vi "Main.vi"() -> ()   [LabVIEW 2014]
uses:
  Goomba Direction.ctl
panel:
  out "Time":i32
  out "Score":i32
  in  "?":bool
  out "?":picture
  in  "Start Game":bool
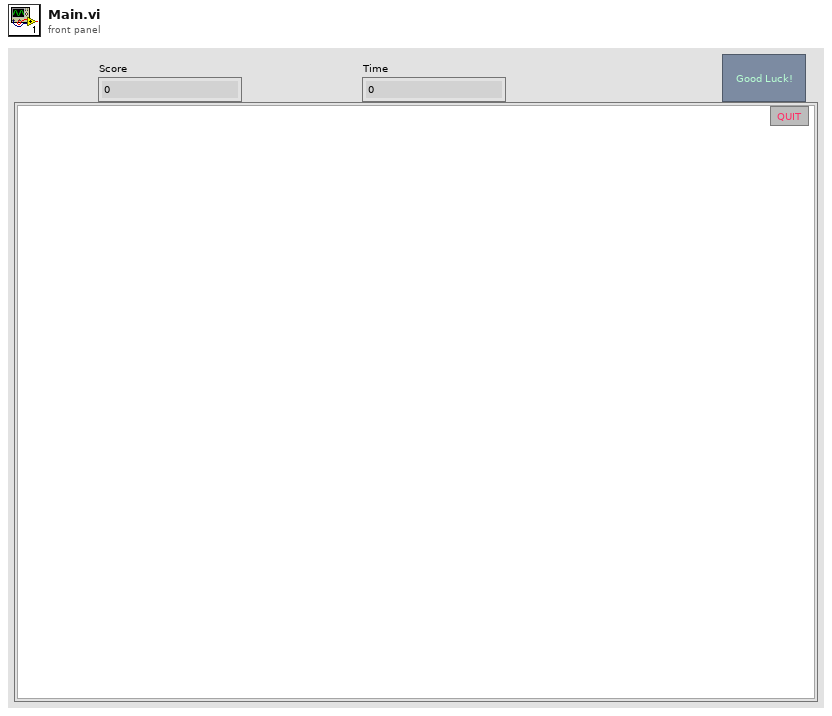
[diagram p1: front panel]
types:
  T1 = typedef "Goomba Direction.ctl" = enum16{"Left", "Right"}
  T2 = typedef "eventvkey.ctl" = enum16{"ASCII", "Enter", "Return", "Shift", "Ctrl", "Alt", "Cmd", "Opt", "Caps", "NumLock", "Clear", "Break", "Up", "Down", "Left", "Right", "Insert", "Delete", "Home", "End", "PageUp", "PageDown", "Escape", "Help", "Pause", "ScrollLock", "F1", "F2", "F3", "F4", "F5", "F6", "F7", "F8", "F9", "F10", "F11", "F12", "F13", "F14", "F15", "F16", "F17", "F18", "F19", "F20", "F21", "F22", "F23", "F24", "Play", "VolumeUp", "VolumeDown", "Mute", "Two Byte Char"}
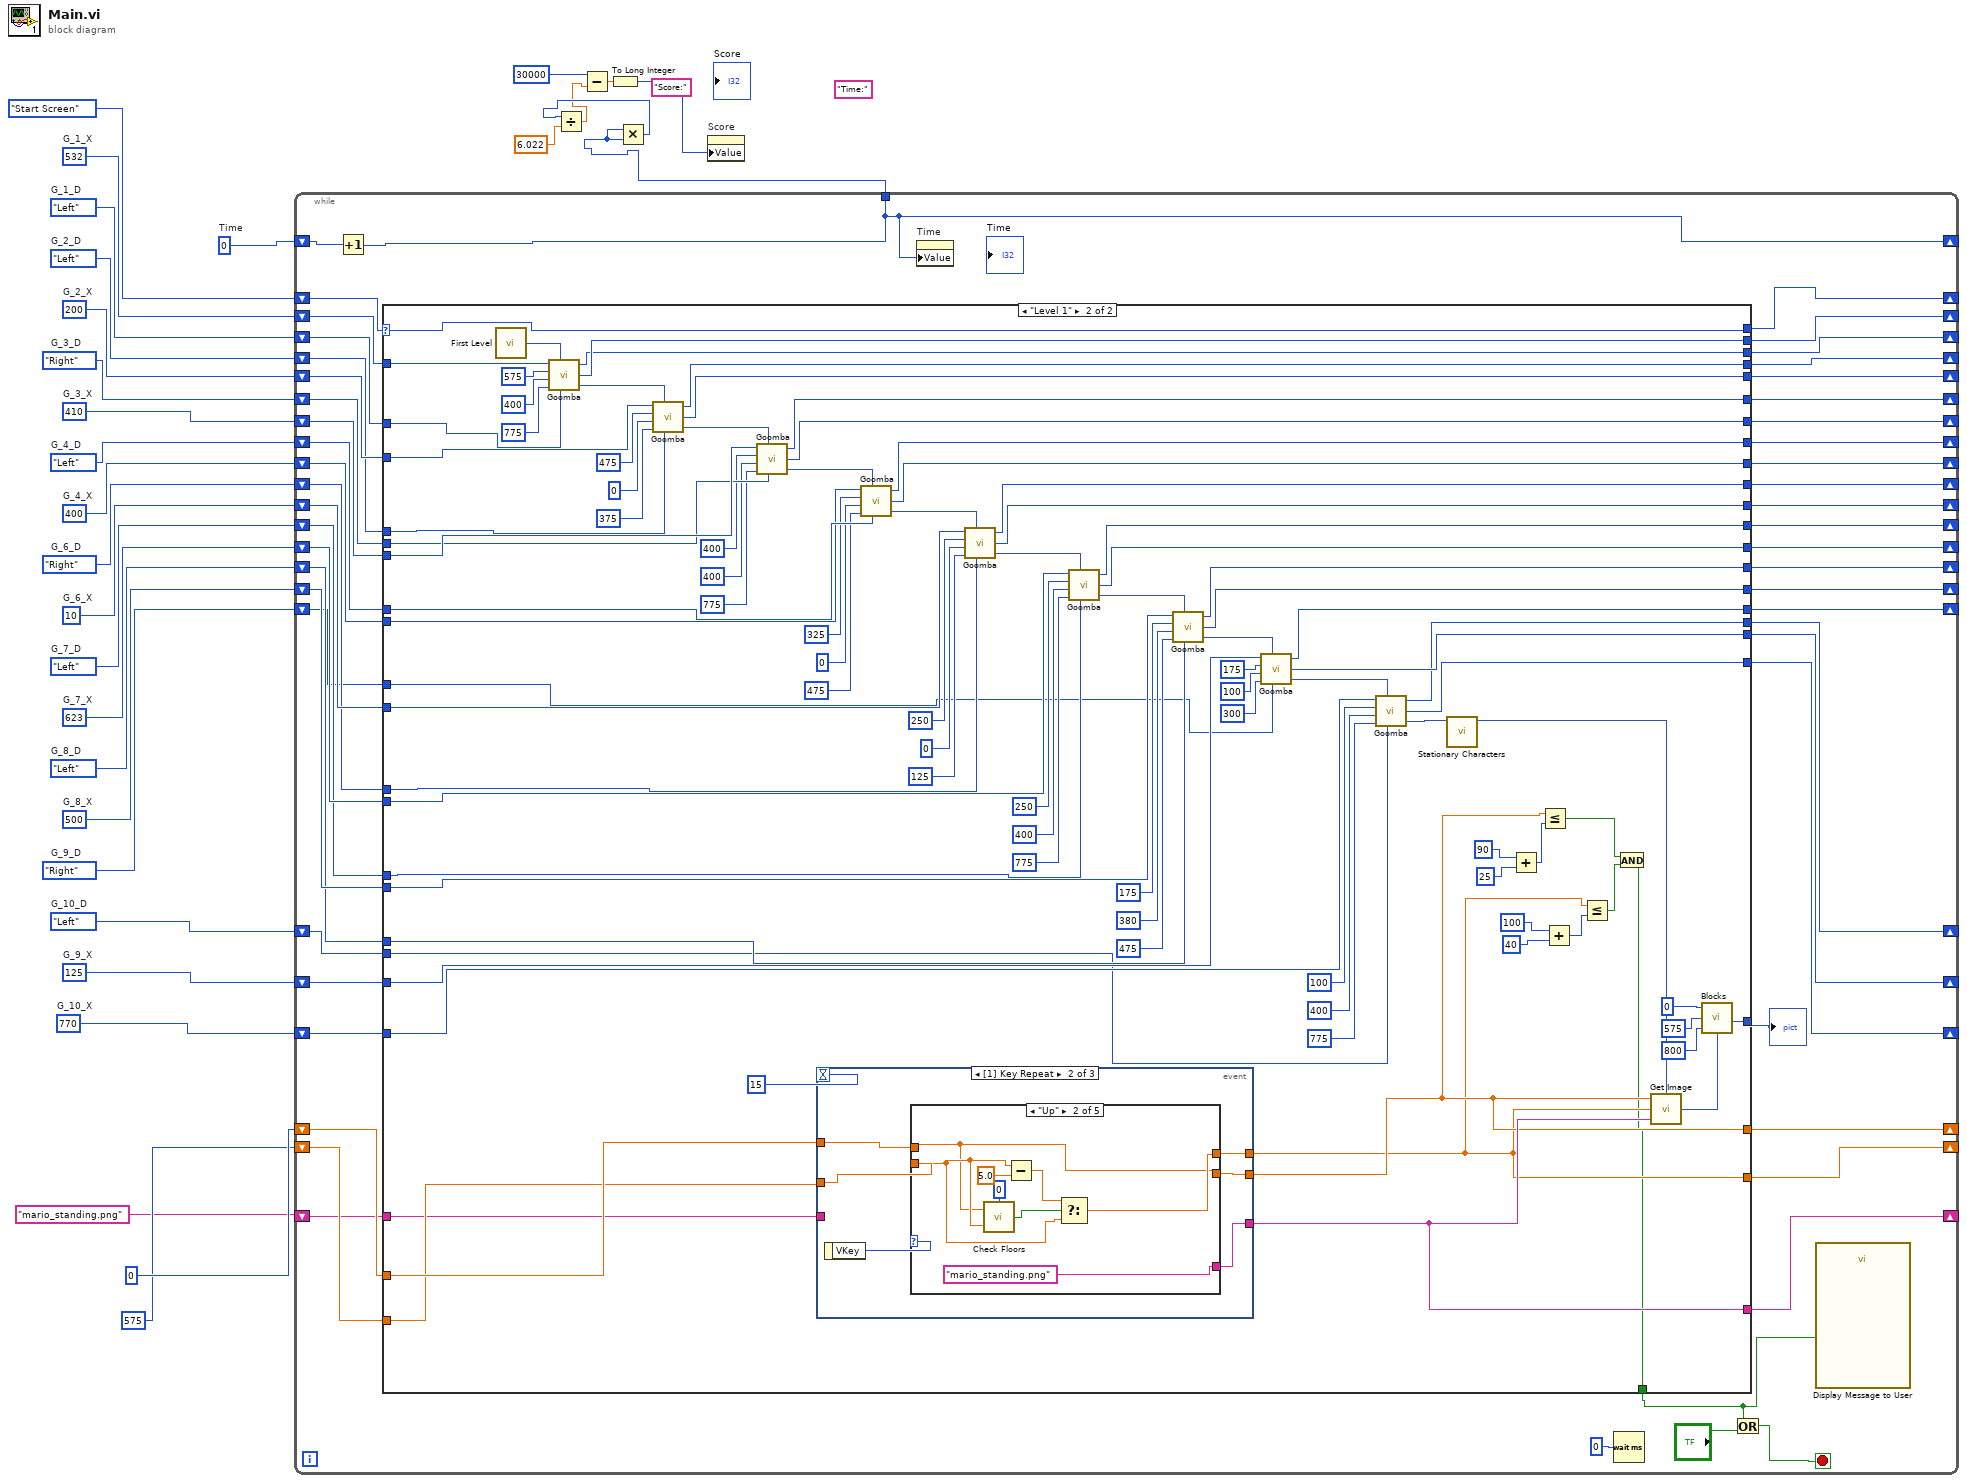
[diagram p0: block diagram]
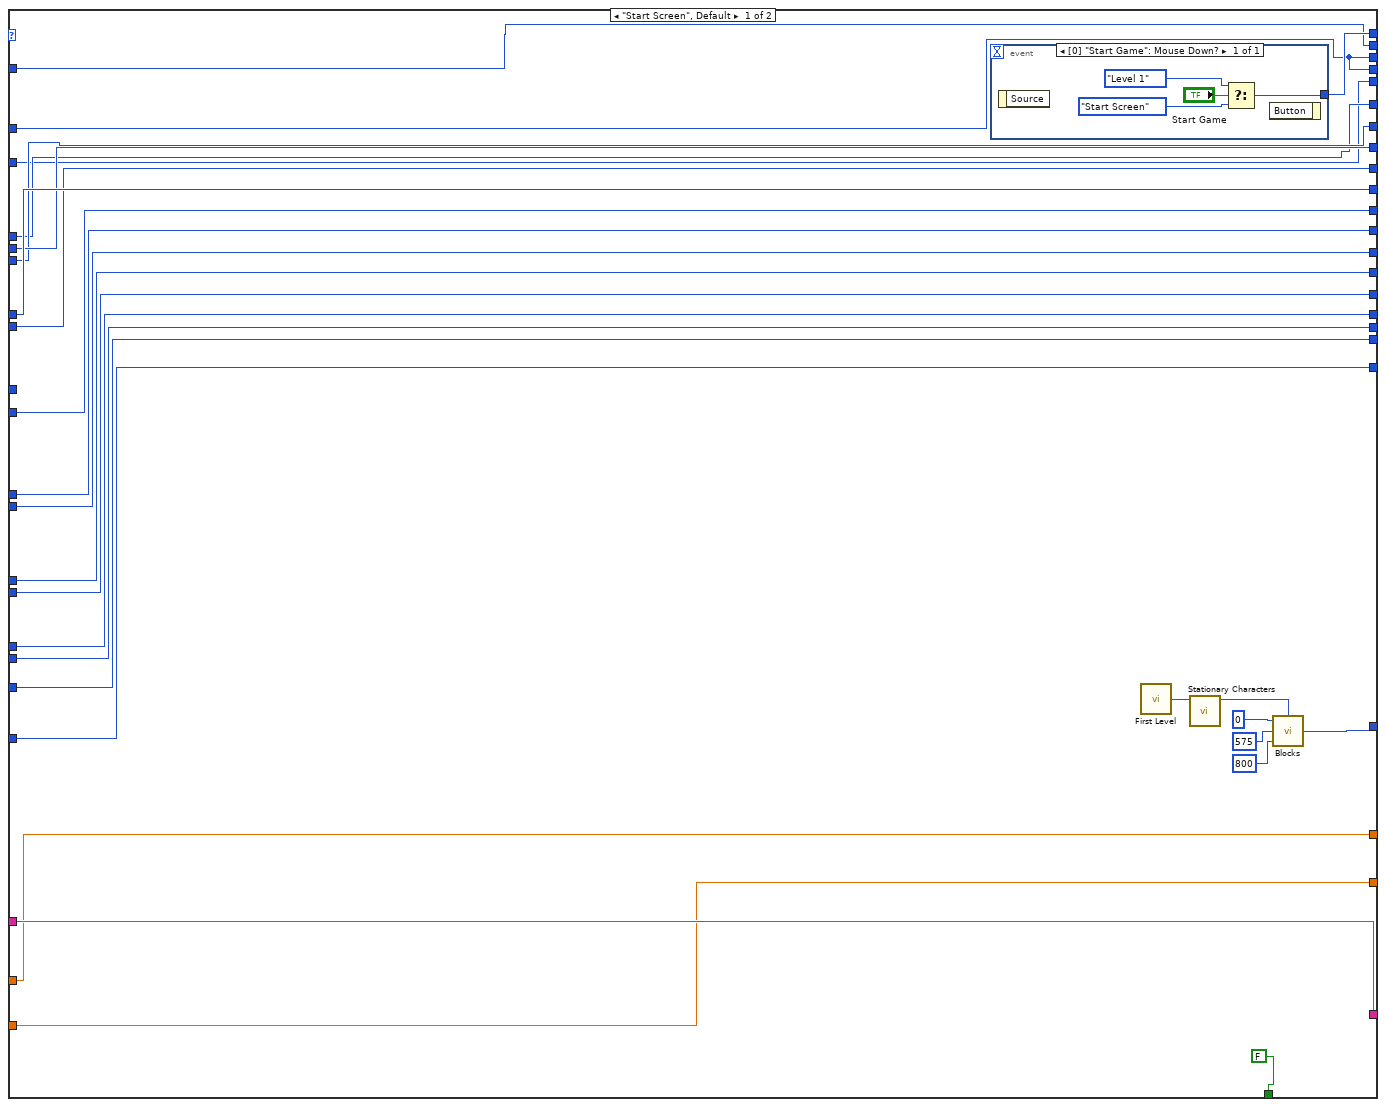
[diagram p2: hidden frame]
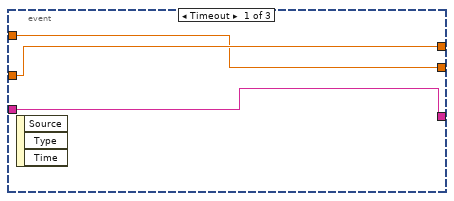
[diagram p3: hidden frame]
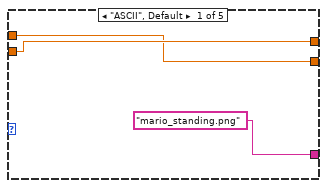
[diagram p4: hidden frame]
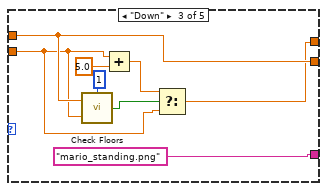
[diagram p5: hidden frame]
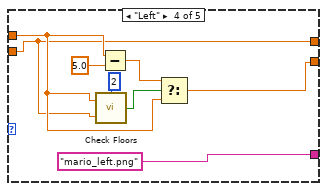
[diagram p6: hidden frame]
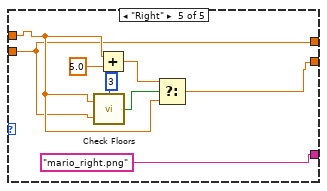
[diagram p7: hidden frame]
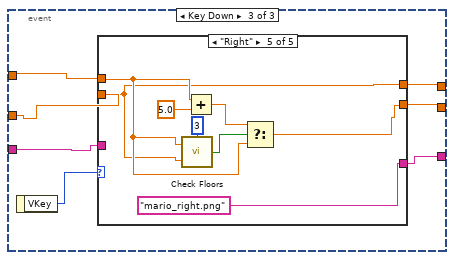
[diagram p8: hidden frame]
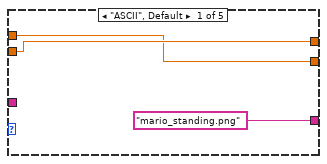
[diagram p9: hidden frame]
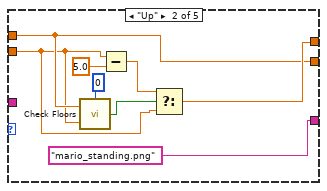
[diagram p10: hidden frame]
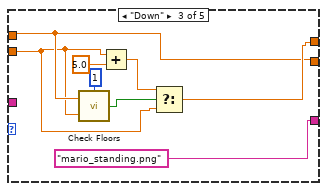
[diagram p11: hidden frame]
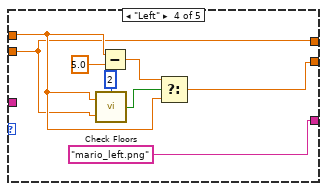
[diagram p12: hidden frame]
diagram:
  (unwired) "Time:" ("gfhgfh")
  (unwired) "Score:"
  w8 = 0  # Time
  w12 = Goomba_Direction."Right"  # G_9_D
  w13 = 125  # G_9_X
  w15 = Goomba_Direction."Left"  # G_8_D
  w14 = 500  # G_8_X
  w19 = Goomba_Direction."Left"  # G_7_D
  w18 = 623  # G_7_X
  w17 = Goomba_Direction."Right"  # G_6_D
  w21 = 10  # G_6_X
  w16 = Goomba_Direction."Left"  # G_10_D
  w22 = 770  # G_10_X
  w20 = Goomba_Direction."Left"  # G_4_D
  w23 = 400  # G_4_X
  w24 = Goomba_Direction."Right"  # G_3_D
  w25 = 410  # G_3_X
  w26 = Goomba_Direction."Left"  # G_2_D
  w27 = 200  # G_2_X
  w28 = Goomba_Direction."Left"  # G_1_D
  w29 = 532  # G_1_X
  n1 = while {
    shift-right: [w37] -> _
    shift-left: enum16{"Start Screen", "Level 1"}."Start Screen" ("Level 2") -> [w38]
    shift-right: [w79] -> _
    shift-left: w29 -> [w80]
    shift-right: [w78] -> _
    shift-left: w28 -> [w77]
    shift-right: [w72] -> _
    shift-left: w26 -> [w75]
    shift-right: [w71] -> _
    shift-left: w27 -> [w76]
    shift-right: [w70] -> _
    shift-left: w24 -> [w73]
    shift-right: [w69] -> _
    shift-left: w25 -> [w74]
    shift-right: [w68] -> _
    shift-left: w20 -> [w57]
    shift-right: [w67] -> _
    shift-left: w23 -> [w56]
    shift-right: [w55] -> _
    shift-left: w17 -> [w63]
    shift-right: [w54] -> _
    shift-left: w21 -> [w64]
    shift-right: [w53] -> _
    shift-left: w19 -> [w61]
    shift-right: [w52] -> _
    shift-left: w18 -> [w62]
    shift-right: [w51] -> _
    shift-left: w15 -> [w59]
    shift-right: [w50] -> _
    shift-left: w14 -> [w60]
    shift-right: [w49] -> _
    shift-left: w12 -> [w31]
    shift-right: [w48] -> _
    shift-left: w13 -> [w58]
    shift-right: [w47] -> _
    shift-left: w16 -> [w65]
    shift-right: [w46] -> _
    shift-left: w22 -> [w66]
    shift-right: [w45] -> _
    shift-left: "mario_standing.png" -> [w42]
    shift-right: [w40] -> _
    shift-left: 0 -> [w44]
    shift-right: [w41] -> _
    shift-left: 575 -> [w43]
    shift-right: [w32] -> _
    shift-left: w8 -> [w39]
    tunnel: [w32] -> w1
    stop <- w34 stop-if-true
    n2 = Increment(x=w39) -> (x+1=w32:i32)
    n3 = case shown="\"Level 1\"" w38 {
      selector: w38 -> [_ w116]
      tunnel: [w104 w116] -> w37
      tunnel: [w103 w204] -> w35
      tunnel: w80 -> [w88 w203]
      tunnel: [w88 w202] -> w79
      tunnel: [w87 w201] -> w78
      tunnel: w77 -> [w87 w188]
      tunnel: w76 -> [w86 w186]
      tunnel: w75 -> [w89 w185]
      tunnel: w74 -> [w90 w184]
      tunnel: w73 -> [w91 w183]
      tunnel: [w87 w182] -> w72
      tunnel: [w86 w181] -> w71
      tunnel: [w89 w174] -> w70
      tunnel: [w90 w173] -> w69
      tunnel: [w91 w172] -> w68
      tunnel: [w92 w171] -> w67
      tunnel: w66 -> [w102 w161]
      tunnel: w65 -> [w101 w160]
      tunnel: w64 -> [w94 w170]
      tunnel: w63 -> [w95 w169]
      tunnel: w62 -> [w96 w168]
      tunnel: w61 -> [w97 w167]
      tunnel: w60 -> [w98 w166]
      tunnel: w59 -> [w99 w165]
      tunnel: w58 -> [w100 w164]
      tunnel: w57 -> [w93 w163]
      tunnel: w56 -> [w92 w162]
      tunnel: [w93 w159] -> w55
      tunnel: [w94 w158] -> w54
      tunnel: [w95 w139] -> w53
      tunnel: [w96 w138] -> w52
      tunnel: [w97 w137] -> w51
      tunnel: [w98 w136] -> w50
      tunnel: [w99 w135] -> w49
      tunnel: [w100 w134] -> w48
      tunnel: [w101 w133] -> w47
      tunnel: [w102 w132] -> w46
      tunnel: [w85 w130] -> w45
      tunnel: w44 -> [w84 w129]
      tunnel: w43 -> [w83 w128]
      tunnel: w42 -> [w85 w127]
      tunnel: [w83 w119] -> w41
      tunnel: [w84 w123] -> w40
      tunnel: [FALSE w115] -> w33
      tunnel: w31 -> [_ w114]
      frame "Start Screen", Default {
        n4 = event shown="[0] \"Start Game\": Mouse Down?" {
          selector: _ -> [_]
          dyn-events: _ -> [_]
          timeout: _ -> [_]
          tunnel: [w111] -> w104
          event "Start Game": Mouse Down? {
            n5 = event-data() -> ()  [unwired: 1 in, 1 out]
            n6 = Select(t=enum16{"Start Screen", "Level 1"}."Level 1" ("Level 2"), s="Start Game", f=enum16{"Start Screen", "Level 1"}."Start Screen" ("Level 2")) -> (s? t:f=w111:enum16{"Start Screen", "Level 1"})
            n7 = event-data() -> ()  [unwired: 2 in, 1 out]
          }
        }
        n8 = call "First Level.vi"() -> ("2D Picture"=w105:picture)
        n9 = call "Stationary Characters.vi"("Main Picture in"=w105) -> ("Main Picture out"=w106:picture)  [unwired: 10 in]
        n10 = call "Blocks.vi"("Input Picture"=w106, "Width"=i16 800, "Origin Y"=i16 575, "Origin X"=i16 0) -> (0:w103:picture)
      }
      frame "Level 1" {
        n11 = call "First Level.vi"() -> ("2D Picture"=w205:picture)
        n12 = call "Goomba.vi"("X Init"=w203, "Picture In"=w205, "Y Init"=575, "Left Bound"=400, "Dir In"=w188, "Right Bound"=775) -> ("Dir Out"=w201:T1, "Pos Out"=w202:i32, "Main Picture"=w196:picture)
        n13 = call "Goomba.vi"("X Init"=w186, "Picture In"=w196, "Y Init"=475, "Left Bound"=0, "Dir In"=w185, "Right Bound"=375) -> ("Dir Out"=w182:T1, "Pos Out"=w181:i32, "Main Picture"=w189:picture)
        n14 = call "Goomba.vi"("X Init"=w184, "Picture In"=w189, "Y Init"=400, "Left Bound"=400, "Dir In"=w183, "Right Bound"=775) -> ("Dir Out"=w174:T1, "Pos Out"=w173:i32, "Main Picture"=w190:picture)
        n15 = event shown="[1] Key Repeat" {
          selector: _ -> [_ _ _]
          dyn-events: _ -> [_ _ _]
          timeout: 15 -> [_ _ _]
          tunnel: [w210 w213 w258] -> w130
          tunnel: w129 -> [w211 w217 w260]
          tunnel: w128 -> [w212 w216 w259]
          tunnel: [w211 w215 w257] -> w123
          tunnel: [w212 w214 w256] -> w119
          tunnel: w127 -> [w210 _ w254]
          event Timeout {
            n16 = event-data() -> ()  [unwired: 1 in, 3 out]
          }
          event Key Repeat {
            n17 = event-data() -> ("VKey"=w218:T2)  [unwired: 1 in]
            n18 = case shown="\"Up\"" w218 {
              tunnel: ["mario_standing.png" "mario_standing.png" "mario_standing.png" "mario_left.png" "mario_right.png"] -> w213
              tunnel: w217 -> [w219 w223 w235 w240 w249]
              tunnel: w216 -> [w220 w225 w230 w239 w247]
              tunnel: [w220 w224 w232 w239 w247] -> w214
              tunnel: [w219 w223 w235 w242 w248] -> w215
              frame "ASCII", Default {
              }
              frame "Up" {
                n19 = call "Check Floors.vi"("Direction"=0, "Bottom"=w225, "Left"=w223) -> ("Boolean"=w227:bool)
                n20 = Subtract(x=w225, y=5.0) -> (x-y=w226:dbl)
                n21 = Select(t=w226, s=w227, f=w225) -> (s? t:f=w224:dbl)
              }
              frame "Down" {
                n22 = call "Check Floors.vi"("Direction"=1, "Bottom"=w230, "Left"=w235) -> ("Boolean"=w234:bool)
                n23 = Add(x=w230, y=5.0) -> (x+y=w233:dbl)
                n24 = Select(t=w233, s=w234, f=w230) -> (s? t:f=w232:dbl)
              }
              frame "Left" {
                n25 = call "Check Floors.vi"("Direction"=2, "Bottom"=w239, "Left"=w240) -> ("Boolean"=w241:bool)
                n26 = Subtract(x=w240, y=5.0) -> (x-y=w243:dbl)
                n27 = Select(t=w243, s=w241, f=w240) -> (s? t:f=w242:dbl)
              }
              frame "Right" {
                n28 = call "Check Floors.vi"("Direction"=3, "Bottom"=w247, "Left"=w249) -> ("Boolean"=w250:bool)
                n29 = Add(x=w249, y=5.0) -> (x+y=w251:dbl)
                n30 = Select(t=w251, s=w250, f=w249) -> (s? t:f=w248:dbl)
              }
            }
          }
          event Key Down {
            n31 = event-data() -> ("VKey"=w255:T2)  [unwired: 1 in]
            n32 = case shown="\"Right\"" w255 {
              tunnel: ["mario_standing.png" "mario_standing.png" "mario_standing.png" "mario_left.png" "mario_right.png"] -> w258
              tunnel: w260 -> [w261 w266 w274 w283 w291]
              tunnel: w259 -> [w262 w265 w273 w282 w290]
              tunnel: [w262 w267 w275 w282 w290] -> w256
              tunnel: [w261 w266 w274 w281 w289] -> w257
              tunnel: w254 -> [_ _ _ _ _]
              frame "ASCII", Default {
              }
              frame "Up" {
                n33 = call "Check Floors.vi"("Direction"=0, "Bottom"=w265, "Left"=w266) -> ("Boolean"=w269:bool)
                n34 = Subtract(x=w265, y=5.0) -> (x-y=w268:dbl)
                n35 = Select(t=w268, s=w269, f=w265) -> (s? t:f=w267:dbl)
              }
              frame "Down" {
                n36 = call "Check Floors.vi"("Direction"=1, "Bottom"=w273, "Left"=w274) -> ("Boolean"=w277:bool)
                n37 = Add(x=w273, y=5.0) -> (x+y=w276:dbl)
                n38 = Select(t=w276, s=w277, f=w273) -> (s? t:f=w275:dbl)
              }
              frame "Left" {
                n39 = call "Check Floors.vi"("Direction"=2, "Bottom"=w282, "Left"=w283) -> ("Boolean"=w284:bool)
                n40 = Subtract(x=w283, y=5.0) -> (x-y=w285:dbl)
                n41 = Select(t=w285, s=w284, f=w283) -> (s? t:f=w281:dbl)
              }
              frame "Right" {
                n42 = call "Check Floors.vi"("Direction"=3, "Bottom"=w290, "Left"=w291) -> ("Boolean"=w292:bool)
                n43 = Add(x=w291, y=5.0) -> (x+y=w293:dbl)
                n44 = Select(t=w293, s=w292, f=w291) -> (s? t:f=w289:dbl)
              }
            }
          }
        }
        n45 = call "Goomba.vi"("X Init"=w162, "Picture In"=w190, "Y Init"=325, "Left Bound"=0, "Dir In"=w163, "Right Bound"=475) -> ("Dir Out"=w172:T1, "Pos Out"=w171:i32, "Main Picture"=w191:picture)
        n46 = call "Goomba.vi"("X Init"=w170, "Picture In"=w191, "Y Init"=250, "Left Bound"=0, "Dir In"=w169, "Right Bound"=125) -> ("Dir Out"=w159:T1, "Pos Out"=w158:i32, "Main Picture"=w192:picture)
        n47 = call "Goomba.vi"("X Init"=w168, "Picture In"=w192, "Y Init"=250, "Left Bound"=400, "Dir In"=w167, "Right Bound"=775) -> ("Dir Out"=w139:T1, "Pos Out"=w138:i32, "Main Picture"=w193:picture)
        n48 = call "Goomba.vi"("X Init"=w166, "Picture In"=w193, "Y Init"=175, "Left Bound"=380, "Dir In"=w165, "Right Bound"=475) -> ("Dir Out"=w137:T1, "Pos Out"=w136:i32, "Main Picture"=w194:picture)
        n49 = call "Goomba.vi"("X Init"=w164, "Picture In"=w194, "Y Init"=175, "Left Bound"=100, "Dir In"=w114, "Right Bound"=300) -> ("Dir Out"=w135:T1, "Pos Out"=w134:i32, "Main Picture"=w195:picture)
        n50 = call "Goomba.vi"("X Init"=w161, "Picture In"=w195, "Y Init"=100, "Left Bound"=400, "Dir In"=w160, "Right Bound"=775) -> ("Dir Out"=w133:T1, "Pos Out"=w132:i32, "Main Picture"=w187:picture)
        n51 = call "Stationary Characters.vi"("Main Picture in"=w187) -> ("Main Picture out"=w206:picture)  [unwired: 10 in]
        n52 = Add(x=90, y=25) -> (x+y=w124:i32)
        n53 = Less Or Equal?(x=w123, y=w124) -> (x <= y?=w118:bool)
        n54 = Add(x=100, y=40) -> (x+y=w120:i32)
        n55 = Less Or Equal?(x=w119, y=w120) -> (x <= y?=w117:bool)
        n56 = And(x=w118, y=w117) -> (x .and. y?=w115:bool)
        n57 = call "Get Image.vi"("Input Picture"=w206, "String"=w130, "Bottom"=w119, "Left"=w123) -> ("Main Picture"=w200:picture)
        n58 = call "Blocks.vi"("Input Picture"=w200, "Width"=i16 800, "Origin Y"=i16 575, "Origin X"=i16 0) -> (0:w204:picture)
      }
    }
    "?" <- w35
    n59 = property on="Time" class="DigNum (strict)"("Value"=w32) -> ()  [unwired: 2 in, 2 out]
    n60 = Wait (ms)(milliseconds to wait=u32 0) -> ()  [unwired: 1 out]
    n61 = Or(x=w33, y="?") -> (x .or. y?=w34:bool)
    n62 = call "Display Message to User"("Enable"=w33) -> ()  [unwired: 9 in, 2 out]
  }
  n63 = Multiply(x=w1, y=w1) -> (x*y=w4:i32)
  n64 = Divide(x=w4, y=6.022) -> (x/y=w3:dbl)
  n65 = Subtract(x=30000, y=w3) -> (x-y=w6:dbl)
  n66 = To Long Integer(number=w6) -> (32bit integer=w2:i32)
  n67 = property on="Score" class="DigNum (strict)"("Value"=w2) -> ()  [unwired: 2 in, 2 out]
